vi "R-Error.vi"() -> ()   [LabVIEW 2014]
panel:
  in  "-199203001":errorcluster={"status"=TRUE, "code"=-199203001, "source"="出现未定义消息"}
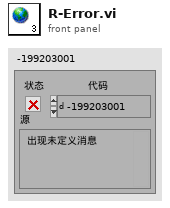
[diagram p1: front panel]
diagram:
